vi "Logging Message Loop.vi"(8 "error in (no error)":errorcluster, 10 "Data Queue":refnum<queue>, 11 "Message Queues":T1) -> (0 "error out":errorcluster)   [LabVIEW 2023, in "Logging.lvlib"]
doc: "The message loop subVI to handle messages pertaining to logging data."
uses:
  Logging.lvlib
  support/Message Queue/All Message Queues.ctl
  support/Message Queue/Message Cluster.ctl
  Logging State.ctl
  support/Message Queue/Enqueue Message (Single).vi
  <vilib>/Utility/error.llb/Error Cluster From Error Code.vi
  <vilib>/ErrorRing/Error Ring.xnode
  support/Message Queue/Message Queue.lvlib
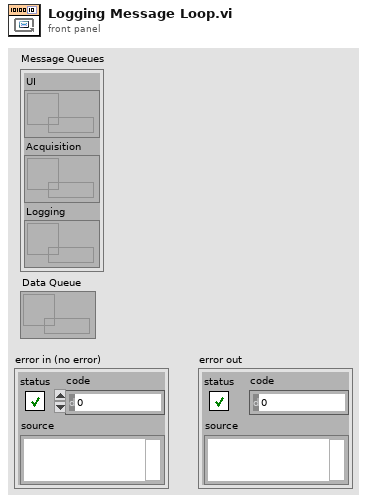
[diagram p1: front panel]
types:
  T1 = typedef "Message Queue.lvlib/All Message Queues.ctl" = cluster{"UI":refnum<queue>, "Acquisition":refnum<queue>, "Logging":refnum<queue>}
  T2 = typedef "Logging.lvlib/Logging State.ctl" = enum16{"Idle", "Logging"}
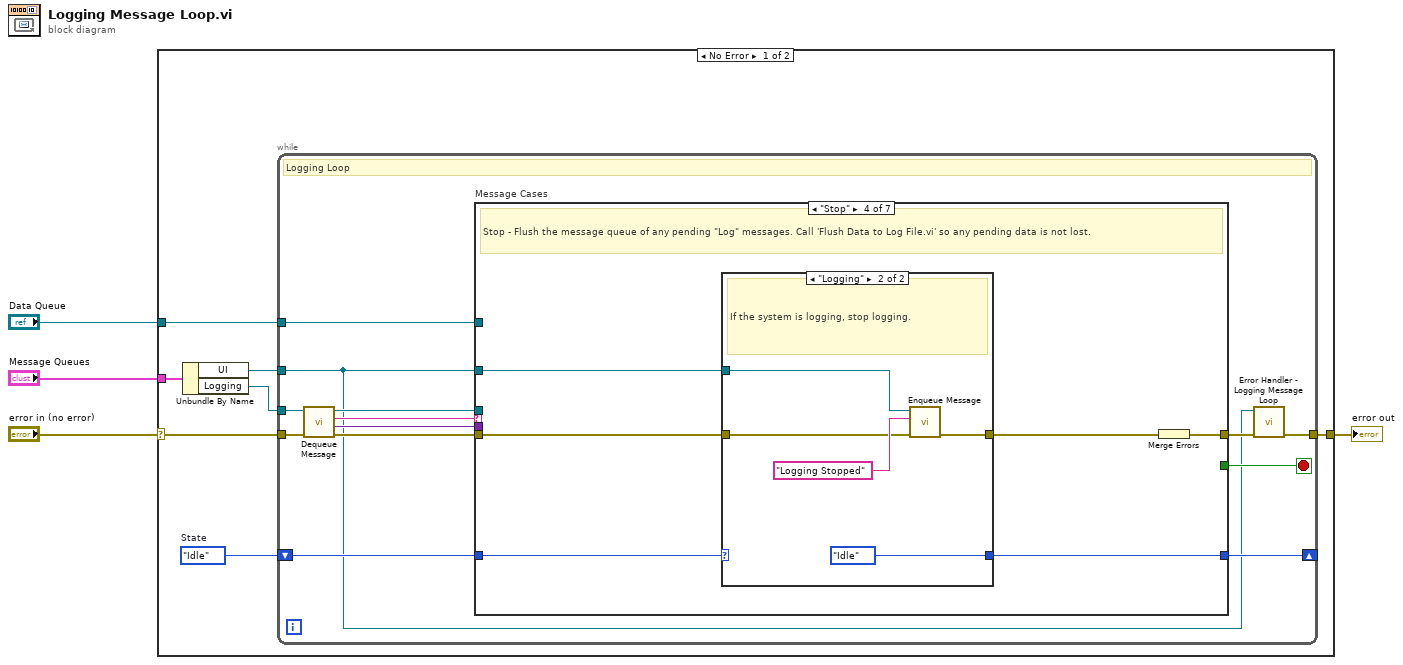
[diagram p0: block diagram]
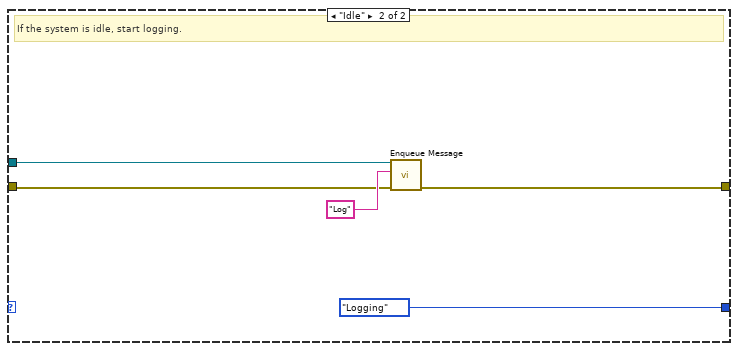
[diagram p4: hidden frame]
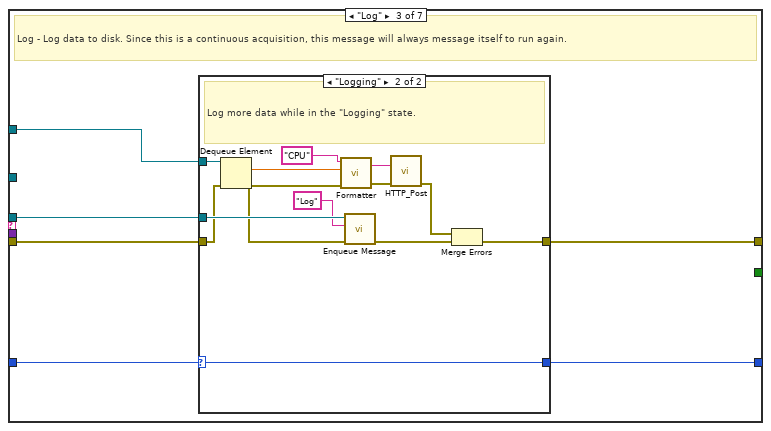
[diagram p5: hidden frame]
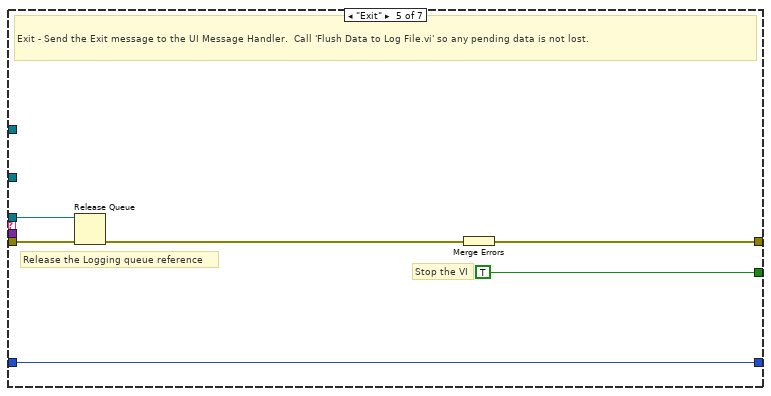
[diagram p8: hidden frame]
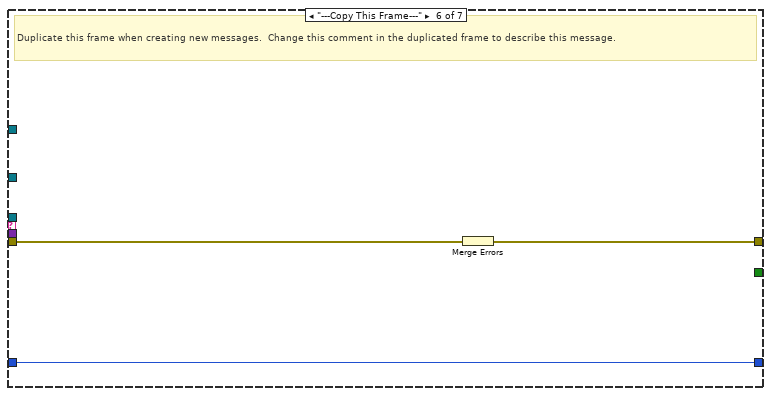
[diagram p9: hidden frame]
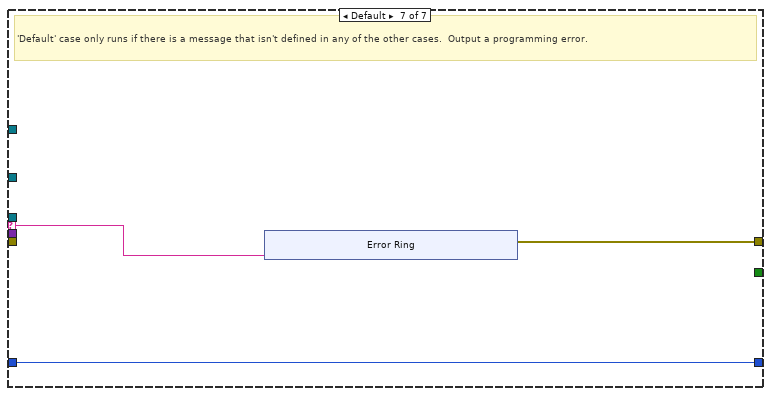
[diagram p10: hidden frame]
diagram:
  n1 = case shown="No Error" "error in (no error)" {
    selector: "error in (no error)" -> [w8 w92]
    tunnel: "Message Queues" -> [w11 _]
    tunnel: [w9 w92] -> w3
    tunnel: "Data Queue" -> [w7 _]
    frame No Error {
      w5 = Logging_State."Idle"  # State
      n2 = Unbundle By Name(w11) -> ("UI"=w6:refnum<queue>, "Logging"=w10:refnum<queue>)
      n3 = while {
        tunnel: w10 -> [w18]
        tunnel: w6 -> [w12]
        tunnel: w7 -> [w17]
        shift-right: [w15] -> _
        shift-left: w5 -> [w16]
        tunnel: w8 -> [w23]
        tunnel: [w14] -> w9
        stop <- w24 stop-if-true
        # "Logging Loop"
        n4 = call "Dequeue Message.vi"("error in (no error)"=w23, "Message Queue"=w18) -> ("error out"=w22:errorcluster, "Message Data"=w20:variant, "Message"=w21:string, "dup Message Queue"=w19:refnum<queue>)  [unwired: 6 in]
        n5 = case "Message Cases" shown="\"Stop\"" w21 {
          selector: w21 -> [_ _ _ _ _ _ w82]
          tunnel: w19 -> [_ w30 w43 _ w75 _ _]
          tunnel: w22 -> [w26 w29 w41 w63 w76 w81 _]
          tunnel: [w26 w31 w44 w65 w77 w80 w83] -> w13
          tunnel: [_ _ _ _ TRUE _ _] -> w24
          tunnel: w20 -> [_ _ _ _ _ _ _]
          tunnel: w12 -> [_ _ _ w60 _ _ _]
          tunnel: w17 -> [_ _ w42 _ _ _ _]
          tunnel: w16 -> [w25 w28 w40 w62 w73 w79 w84]
          tunnel: [w25 w27 w39 w61 w73 w79 w84] -> w15
          frame "Initialize" {
            # "Initialize - gets called when first launched. Currently a no-op."
          }
          frame "Start" {
            # "Start - Send the \"Log\" message to start logging.  Generate a unique, timestamped TDMS file name based on the Log File Base Path value."
            n6 = case shown="\"Logging\"" w28 {
              selector: w28 -> [w33 _]
              tunnel: [w32 w34] -> w31
              tunnel: w30 -> [_ w36]
              tunnel: w29 -> [w32 w35]
              tunnel: [w33 Logging_State."Logging" ("State")] -> w27
              frame "Logging" {
                # "The system is already logging. Ignore the \"Start\" message."
              }
              frame "Idle" {
                # "If the system is idle, start logging."
                n7 = call-poly "Enqueue Message.vi"("error in (no error)"=w35, "Message"="Log", "Message Queue"=w36) -> ("error out"=w34:errorcluster)  [unwired: 7 in, 1 out]
              }
            }
          }
          frame "Log" {
            # "Log - Log data to disk. Since this is a continuous acquisition, this message will always message itself to run again."
            n8 = case shown="\"Logging\"" w40 {
              selector: w40 -> [w46 w53]
              tunnel: [w45 w59] -> w44
              tunnel: w43 -> [_ w57]
              tunnel: w42 -> [_ w55]
              tunnel: w41 -> [w45 w54]
              tunnel: [w46 w53] -> w39
              frame "Idle" {
                # "Ignore \"Log\" messages when the logging is idle."
              }
              frame "Logging" {
                # "Log more data while in the \"Logging\" state."
                n9 = Dequeue Element(queue=w55, error in (no error)=w54) -> (element=w48:dbl, error out=w51:errorcluster)  [unwired: 1 in, 2 out]
                n10 = call "Formatter.vi"("error in (no error)"=w51, "Variant"=w48, "ID"="CPU") -> ("error out"=w50:errorcluster, "output"=w47:string)  [unwired: 1 in]
                n11 = call-poly "Enqueue Message.vi"("error in (no error)"=w51, "Message"="Log", "Message Queue"=w57) -> ("error out"=w58:errorcluster)  [unwired: 7 in, 1 out]
                n12 = call "HTTP_Post.vi"("data"=w47, "error in (no error)"=w50) -> ("error out"=w52:errorcluster)  [unwired: 5 in, 2 out]
                n13 = Merge Errors(w52, w58) -> (w59:errorcluster)
              }
            }
          }
          frame "Stop" {
            # "Stop - Flush the message queue of any pending \"Log\" messages. Call 'Flush Data to Log File.vi' so any pending data is not lost."
            n14 = case shown="\"Logging\"" w62 {
              selector: w62 -> [w66 _]
              tunnel: [w67 w71] -> w64
              tunnel: w63 -> [w67 w68]
              tunnel: [w66 Logging_State."Idle" ("State")] -> w61
              tunnel: w60 -> [_ w70]
              frame "Idle" {
                # "The system is already idle. Ignore the \"Stop\" message."
              }
              frame "Logging" {
                # "If the system is logging, stop logging."
                n15 = call-poly "Enqueue Message.vi"("error in (no error)"=w68, "Message"="Logging Stopped", "Message Queue"=w70) -> ("error out"=w71:errorcluster)  [unwired: 7 in, 1 out]
              }
            }
            n16 = Merge Errors(w64) -> (w65:errorcluster)
          }
          frame "Exit" {
            # "Release the Logging queue reference"
            # "Stop the VI"
            # "Exit - Send the Exit message to the UI Message Handler.  Call 'Flush Data to Log File.vi' so any pending data is not lost."
            n17 = Release Queue(queue=w75, error in (no error)=w76) -> (error out=w74:errorcluster)  [unwired: 1 in, 2 out]
            n18 = Merge Errors(w74) -> (w77:errorcluster)
          }
          frame "---Copy This Frame---" {
            # "Duplicate this frame when creating new messages.  Change this comment in the duplicated frame to describe this message."
            n19 = Merge Errors(w81) -> (w80:errorcluster)
          }
          frame Default {
            # "'Default' case only runs if there is a message that isn't defined in any of the other cases.  Output a programming error."
            n20 = xnode "Error Ring"("parameter 0"=w82) -> ("error out"=w83:errorcluster)
          }
        }
        n21 = call "Error Handler - Logging Message Loop.vi"("error in (no error)"=w13, "Message Queue"=w12) -> ("dup error in"=w14:errorcluster)  [unwired: 8 in, 1 out]
      }
    }
    frame Error {
    }
  }
  "error out" <- w3
